vi "region-roll parameters-1.vi"() -> ()   [LabVIEW 2009]
panel:
  in  "Calculate 3":bool
  in  "Change_Max Diameter":dbl=108.0
  out "Region 3":dbl format="%_3g"
  out "Lap 3":dbl
  out "Set voltage value 2":dbl format="%_3g"
  out "Voltage difference value 2":dbl format="%_3g"
  in  "Speed-voltage constant 2":dbl=0.01
  out "Min Circular Speed 2":dbl format="%_3g"
  in  "Web Speed 2":dbl=90.0
  in  "Actual Diameter 2":dbl
  out "Max Circular Speed 2":dbl format="%_3g"
  in  "Max Diameter":dbl=108.0
  in  "Min Diameter":dbl=93.0
  in  "Diameter":dbl
  in  "Web Thickness 2":dbl=60.0
  out "Lap 2":dbl
  out "Region 2":dbl format="%_3g"
  out "Output voltage value 2":dbl=0.01 format="%.2g"
  in  "Calculate 2":bool
  in  "Calculate_auto":bool
  in  "Initial Min Diameter":dbl=93.0
  out "Output voltage value":dbl=0.01 format="%.2g"
  out "Set voltage value":dbl format="%_3g"
  out "Voltage difference value":dbl format="%_3g"
  in  "Speed-voltage constant":dbl=0.01
  out "Lap":dbl
  out "Region":dbl format="%_3g"
  in  "Web Thickness":dbl=60.0
  out "Min Circular Speed":dbl format="%_3g"
  out "Max Circular Speed":dbl format="%_3g"
  in  "Web Speed":dbl=90.0
  in  "Total length":dbl
  in  "Calculate":bool
  out "Actual Diameter":dbl
  in  "Change_Min Diameter":dbl=93.0
  # "m"
  # "mm"
  # "mm"
  # "µm"
  # "cm / min"
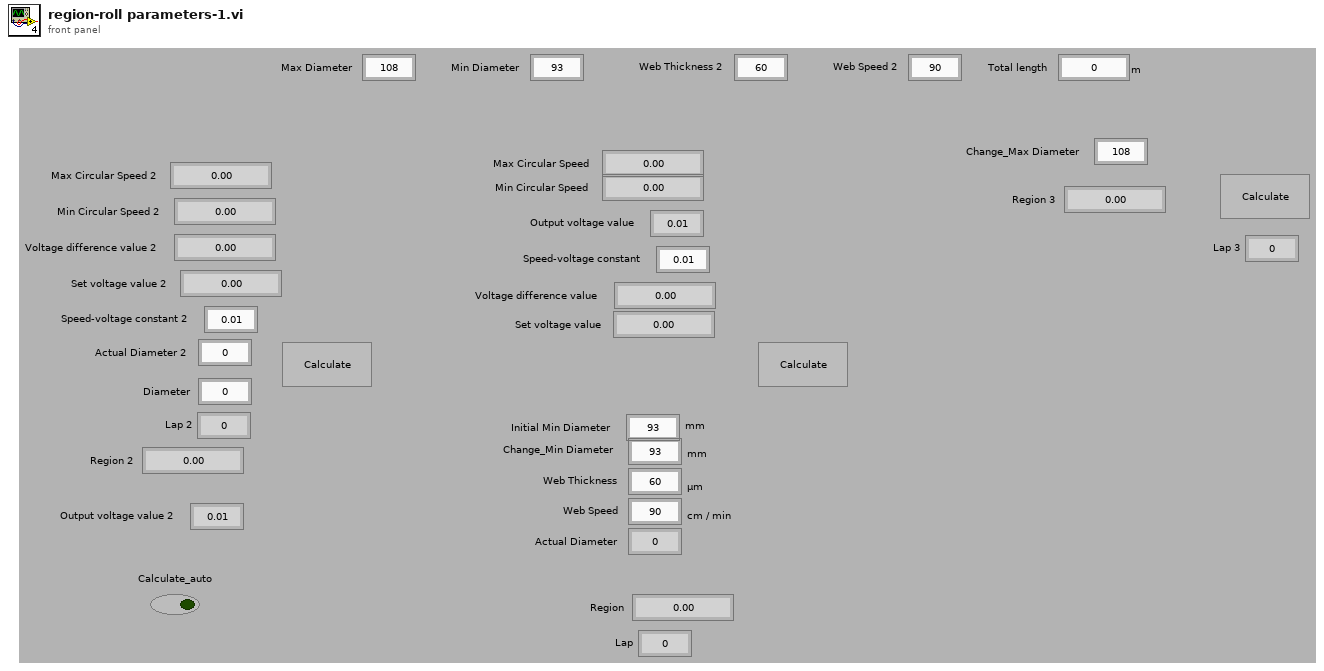
[diagram p1: front panel]
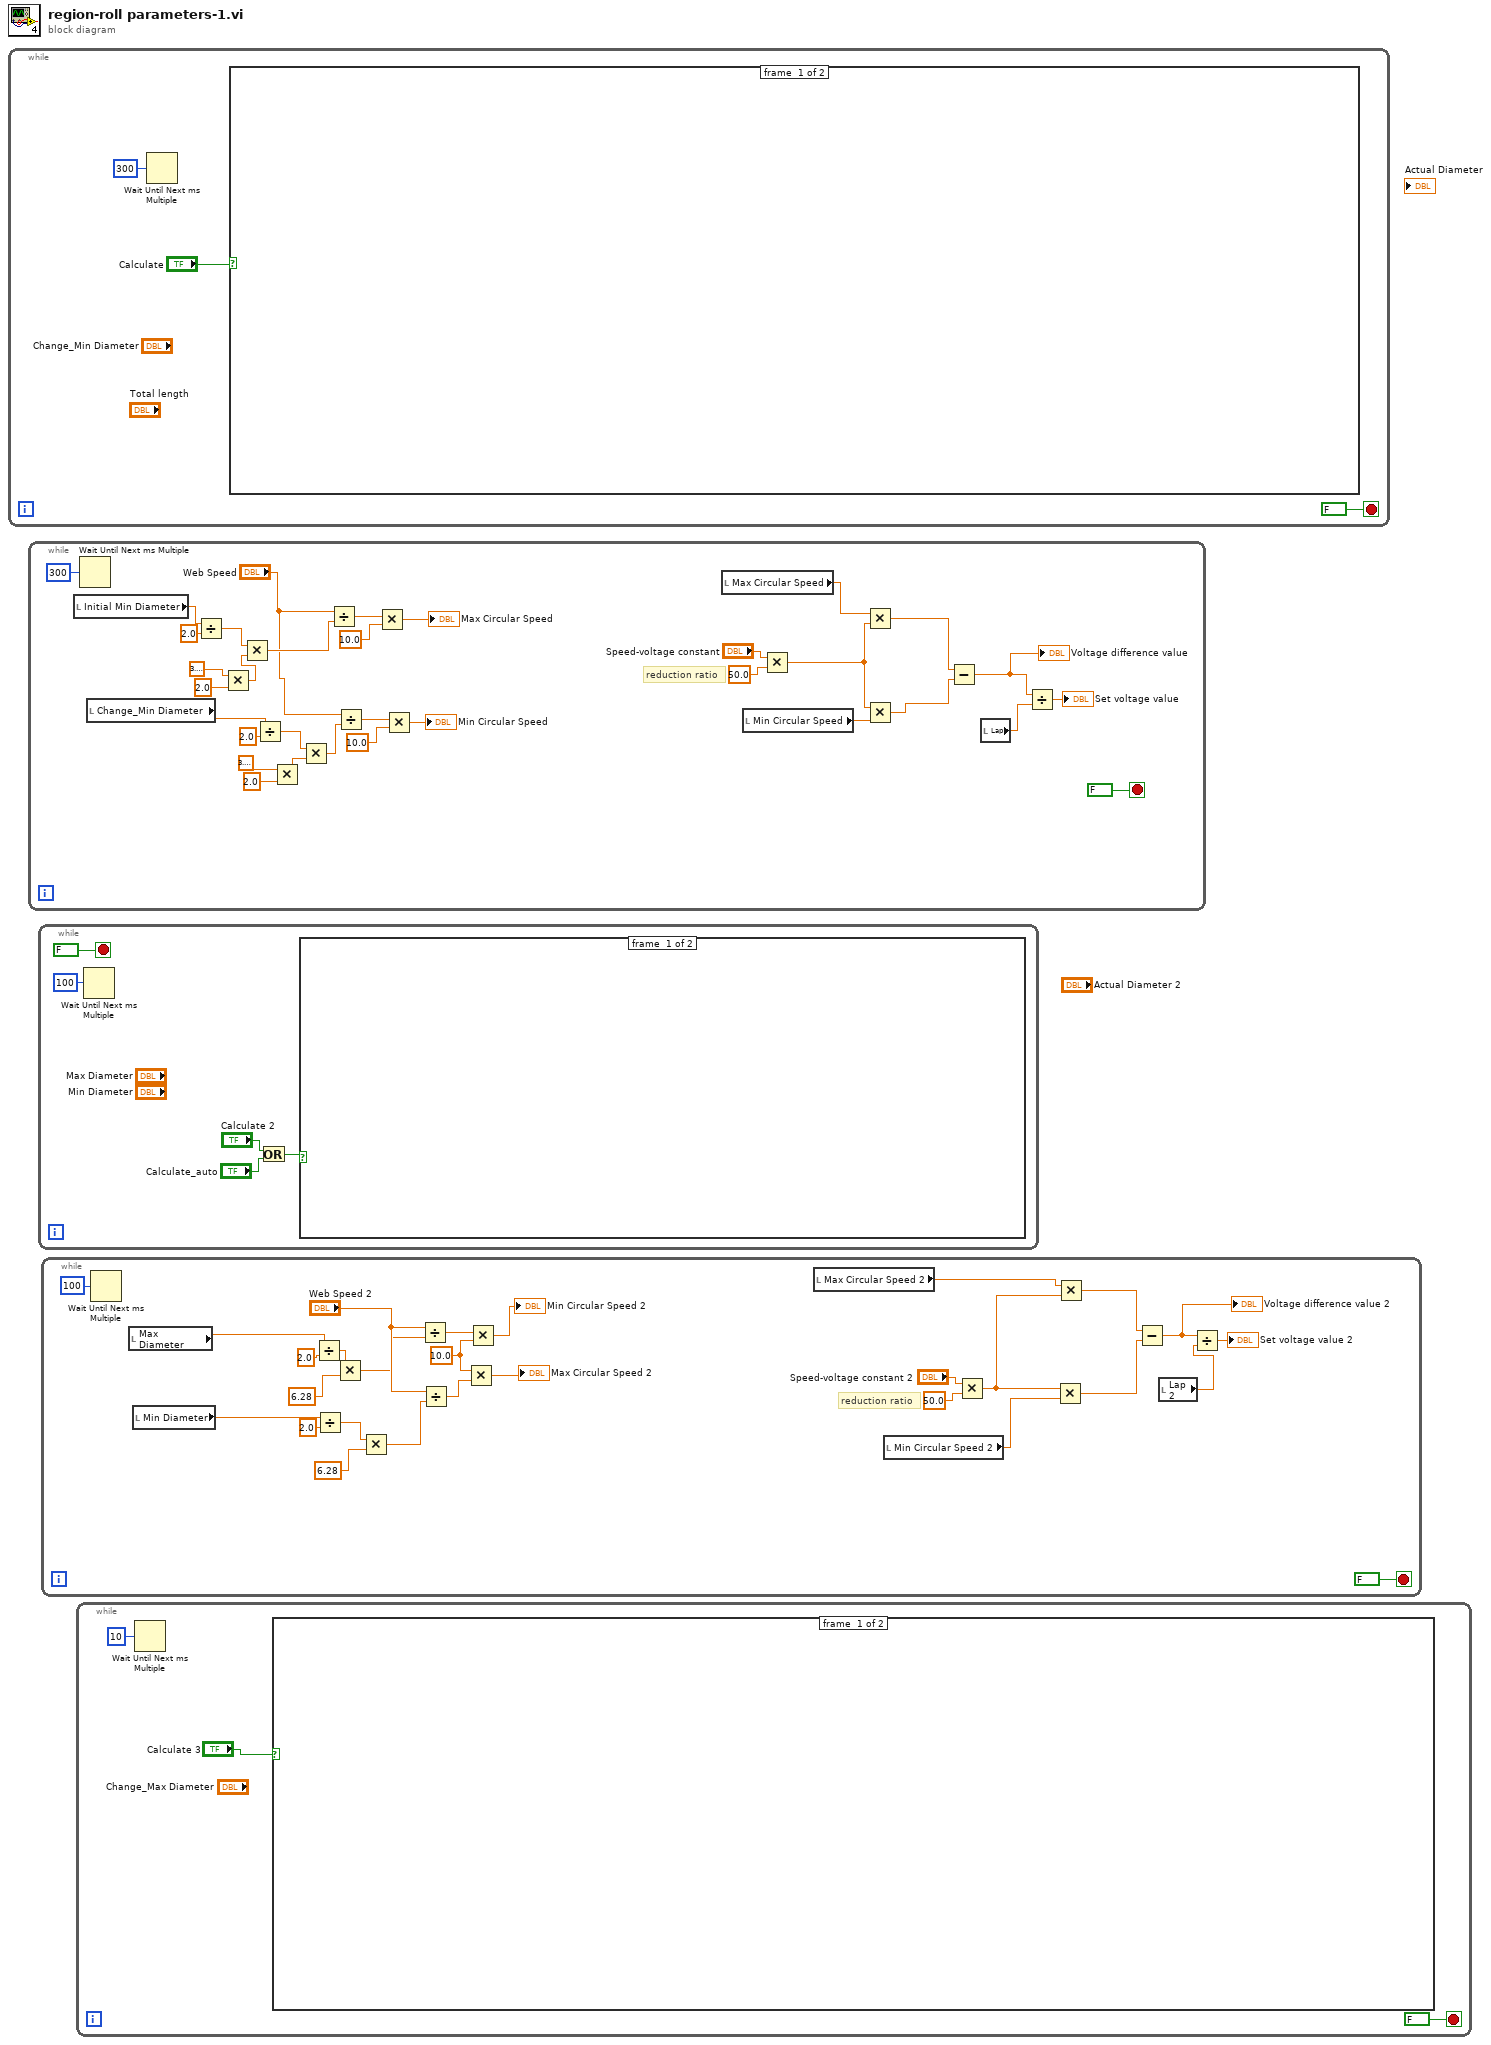
[diagram p0: block diagram]
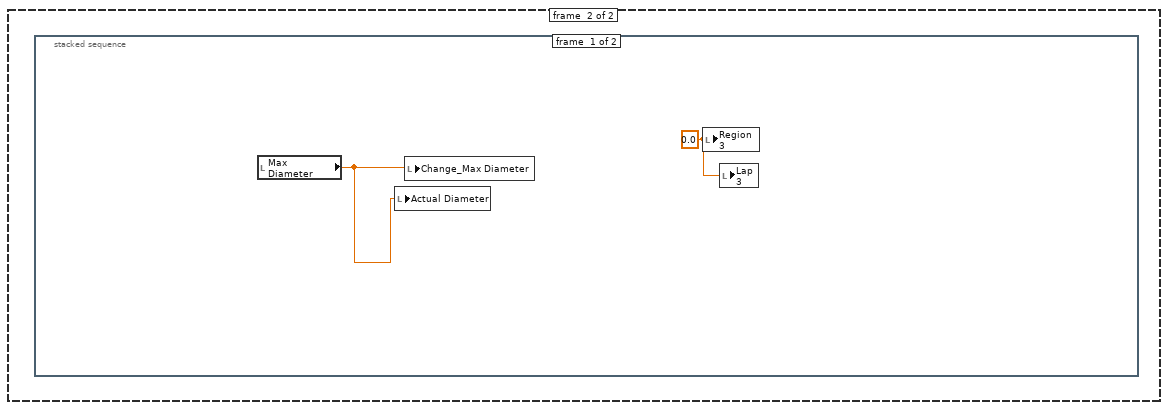
[diagram p2: hidden frame]
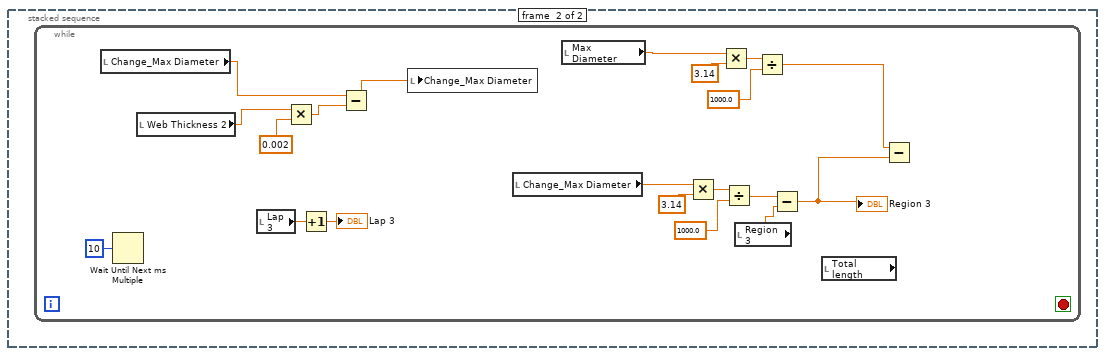
[diagram p3: hidden frame]
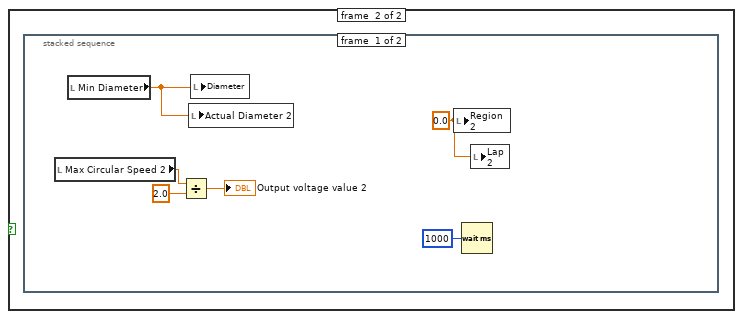
[diagram p4: hidden frame]
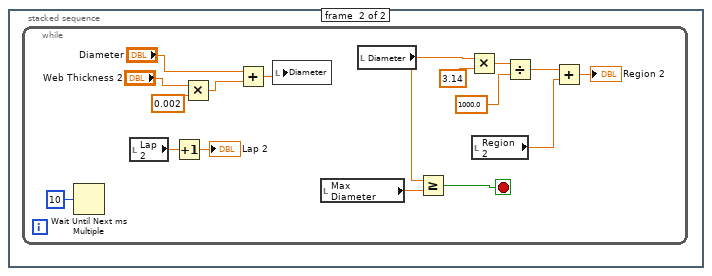
[diagram p5: hidden frame]
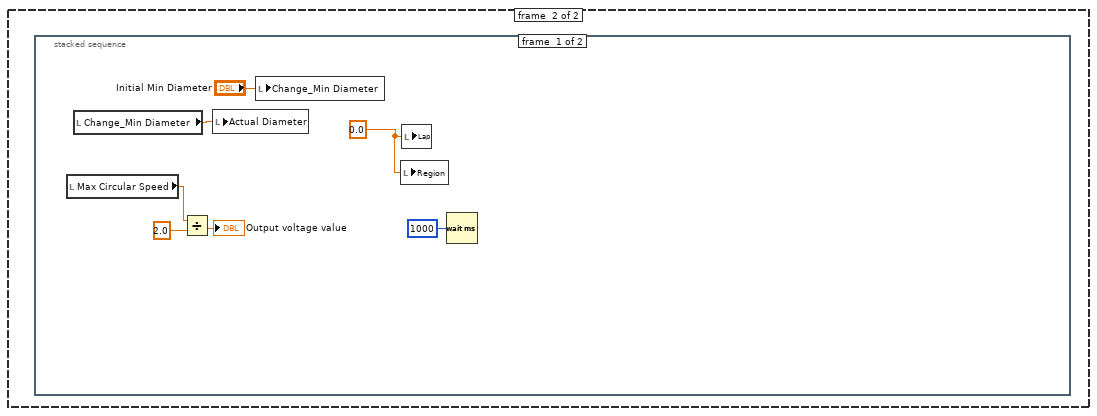
[diagram p6: hidden frame]
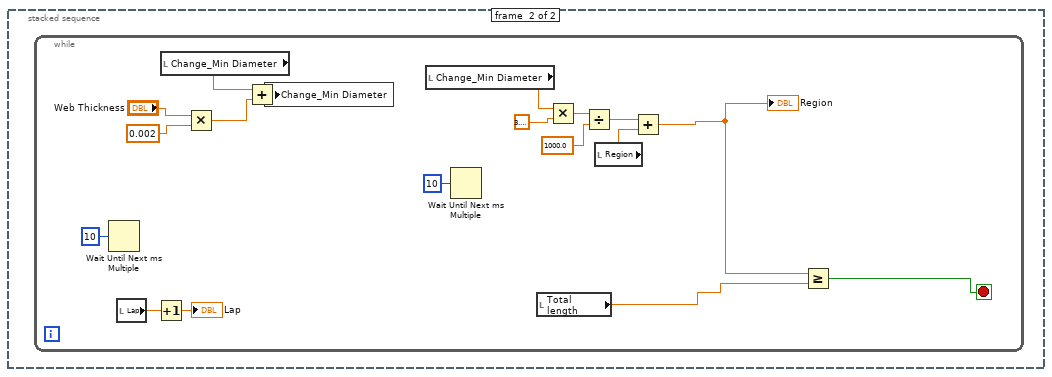
[diagram p7: hidden frame]
diagram:
  n1 = while {
    stop <- FALSE stop-if-true
    n2 = Wait Until Next ms Multiple(millisecond multiple=u32 300) -> ()  [unwired: 1 out]
    n3 = case shown="True" "Calculate" {
      frame #0 {
      }
      frame #1 {
        n4 = stacked-sequence {
          frame #0 {
            w4 = 0.0 ("Lap")
            n5 = local read "Max Circular Speed"() -> (w7:dbl)
            n6 = local read "Change_Min Diameter"() -> (w9:dbl)
            n7 = Divide(x=w7, y=2.0) -> (x/y=→"Output voltage value":dbl)
            n8 = local write "Actual Diameter"(w9) -> ()
            n9 = local write "Change_Min Diameter"("Initial Min Diameter") -> ()
            n10 = local write "Region"(w4) -> ()
            n11 = local write "Lap"(w4) -> ()
            n12 = Wait (ms)(milliseconds to wait=u32 1000) -> ()  [unwired: 1 out]
          }
          frame #1 {
            n13 = while {
              stop <- w20 stop-if-true
              n14 = Wait Until Next ms Multiple(millisecond multiple=u32 10) -> ()  [unwired: 1 out]
              n15 = local read "Lap"() -> (w23:dbl)
              n16 = Increment(x=w23) -> (x+1=→"Lap":dbl)
              n17 = local read "Change_Min Diameter"() -> (w27:dbl)
              n18 = Multiply(x="Web Thickness", y=0.002) -> (x*y=w26:dbl)
              n19 = Add(x=w27, y=w26) -> (x+y=w25:dbl)
              n20 = local write "Change_Min Diameter"(w25) -> ()
              n21 = local read "Change_Min Diameter"() -> (w17:dbl)
              n22 = Wait Until Next ms Multiple(millisecond multiple=u32 10) -> ()  [unwired: 1 out]
              n23 = local read "Total length"() -> (w11:dbl)
              n24 = Multiply(x=w17, y=3.141592653589793) -> (x*y=w18:dbl)
              n25 = Divide(x=w18, y=1000.0) -> (x/y=w19:dbl)
              n26 = local read "Region"() -> (w15:dbl)
              n27 = Add(x=w19, y=w15) -> (x+y=w12:dbl)
              "Region" <- w12
              n28 = Greater Or Equal?(x=w12, y=w11) -> (x >= y?=w20:bool)
            }
          }
        }
      }
    }
  }
  n29 = while {
    stop <- FALSE stop-if-true
    # "reduction ratio"
    n30 = local read "Initial Min Diameter"() -> (w29:dbl)
    n31 = Wait Until Next ms Multiple(millisecond multiple=u32 300) -> ()  [unwired: 1 out]
    n32 = local read "Change_Min Diameter"() -> (w30:dbl)
    n33 = Divide(x=w29, y=2.0) -> (x/y=w59:dbl)
    n34 = Multiply(x=3.141592653589793, y=2.0) -> (x*y=w45:dbl)
    n35 = Multiply(x=w59, y=w45) -> (x*y=w56:dbl)
    n36 = Divide(x=w30, y=2.0) -> (x/y=w51:dbl)
    n37 = Multiply(x=3.141592653589793, y=2.0) -> (x*y=w42:dbl)
    n38 = Multiply(x=w51, y=w42) -> (x*y=w54:dbl)
    n39 = Divide(x="Web Speed", y=w56) -> (x/y=w58:dbl)
    n40 = Divide(x="Web Speed", y=w54) -> (x/y=w52:dbl)
    n41 = Multiply(x=w58, y=10.0) -> (x*y=→"Max Circular Speed":dbl)
    n42 = Multiply(x=w52, y=10.0) -> (x*y=→"Min Circular Speed":dbl)
    n43 = local read "Max Circular Speed"() -> (w38:dbl)
    n44 = local read "Min Circular Speed"() -> (w37:dbl)
    n45 = Multiply(x="Speed-voltage constant", y=50.0) -> (x*y=w39:dbl)
    n46 = Multiply(x=w38, y=w39) -> (x*y=w36:dbl)
    n47 = Multiply(x=w39, y=w37) -> (x*y=w35:dbl)
    n48 = Subtract(x=w36, y=w35) -> (x-y=w32:dbl)
    "Voltage difference value" <- w32
    n49 = local read "Lap"() -> (w33:dbl)
    n50 = Divide(x=w32, y=w33) -> (x/y=→"Set voltage value":dbl)
  }
  n51 = while {
    stop <- FALSE stop-if-true
    n52 = Wait Until Next ms Multiple(millisecond multiple=u32 100) -> ()  [unwired: 1 out]
    n53 = Or(x="Calculate 2", y="Calculate_auto") -> (x .or. y?=w64:bool)
    n54 = case shown="True" w64 {
      frame #0 {
      }
      frame #1 {
        n55 = stacked-sequence {
          frame #0 {
            w71 = 0.0 ("Region")
            n56 = local read "Max Circular Speed 2"() -> (w68:dbl)
            n57 = local read "Min Diameter"() -> (w67:dbl)
            n58 = Divide(x=w68, y=2.0) -> (x/y=→"Output voltage value 2":dbl)
            n59 = local write "Actual Diameter 2"(w67) -> ()
            n60 = local write "Diameter"(w67) -> ()
            n61 = local write "Region 2"(w71) -> ()
            n62 = Wait (ms)(milliseconds to wait=u32 1000) -> ()  [unwired: 1 out]
            n63 = local write "Lap 2"(w71) -> ()
          }
          frame #1 {
            n64 = while {
              stop <- w76 stop-if-true
              n65 = Wait Until Next ms Multiple(millisecond multiple=u32 10) -> ()  [unwired: 1 out]
              n66 = local read "Lap 2"() -> (w73:dbl)
              n67 = Increment(x=w73) -> (x+1=→"Lap 2":dbl)
              n68 = Multiply(x="Web Thickness 2", y=0.002) -> (x*y=w87:dbl)
              n69 = Add(x="Diameter", y=w87) -> (x+y=w79:dbl)
              n70 = local write "Diameter"(w79) -> ()
              n71 = local read "Max Diameter"() -> (w78:dbl)
              n72 = local read "Diameter"() -> (w77:dbl)
              n73 = Greater Or Equal?(x=w77, y=w78) -> (x >= y?=w76:bool)
              n74 = Multiply(x=w77, y=3.14) -> (x*y=w81:dbl)
              n75 = local read "Region 2"() -> (w85:dbl)
              n76 = Divide(x=w81, y=1000.0) -> (x/y=w84:dbl)
              n77 = Add(x=w84, y=w85) -> (x+y=→"Region 2":dbl)
            }
          }
        }
      }
    }
  }
  n78 = while {
    stop <- FALSE stop-if-true
    w113 = 10.0 ("y")
    # "reduction ratio"
    n79 = Wait Until Next ms Multiple(millisecond multiple=u32 100) -> ()  [unwired: 1 out]
    n80 = local read "Max Diameter"() -> (w103:dbl)
    n81 = local read "Min Diameter"() -> (w102:dbl)
    n82 = Divide(x=w103, y=2.0) -> (x/y=w108:dbl)
    n83 = Divide(x=w102, y=2.0) -> (x/y=w107:dbl)
    n84 = Multiply(x=w108, y=6.28) -> (x*y=w109:dbl)
    n85 = Multiply(x=w107, y=6.28) -> (x*y=w106:dbl)
    n86 = Divide(x="Web Speed 2", y=w109) -> (x/y=w115:dbl)
    n87 = Divide(x="Web Speed 2", y=w106) -> (x/y=w114:dbl)
    n88 = Multiply(x=w113, y=w114) -> (x*y=→"Max Circular Speed 2":dbl)
    n89 = Multiply(x=w115, y=w113) -> (x*y=→"Min Circular Speed 2":dbl)
    n90 = local read "Max Circular Speed 2"() -> (w99:dbl)
    n91 = local read "Min Circular Speed 2"() -> (w97:dbl)
    n92 = Multiply(x="Speed-voltage constant 2", y=50.0) -> (x*y=w98:dbl)
    n93 = Multiply(x=w98, y=w97) -> (x*y=w93:dbl)
    n94 = Multiply(x=w99, y=w98) -> (x*y=w94:dbl)
    n95 = Subtract(x=w94, y=w93) -> (x-y=w96:dbl)
    "Voltage difference value 2" <- w96
    n96 = local read "Lap 2"() -> (w92:dbl)
    n97 = Divide(x=w96, y=w92) -> (x/y=→"Set voltage value 2":dbl)
  }
  n98 = while {
    stop <- FALSE stop-if-true
    n99 = Wait Until Next ms Multiple(millisecond multiple=u32 10) -> ()  [unwired: 1 out]
    n100 = case shown="True" "Calculate 3" {
      frame #0 {
      }
      frame #1 {
        n101 = stacked-sequence {
          frame #0 {
            w122 = 0.0 ("Region")
            n102 = local read "Max Diameter"() -> (w121:dbl)
            n103 = local write "Actual Diameter"(w121) -> ()
            n104 = local write "Change_Max Diameter"(w121) -> ()
            n105 = local write "Region 3"(w122) -> ()
            n106 = local write "Lap 3"(w122) -> ()
          }
          frame #1 {
            n107 = while {
              stop <- _ stop-if-true
              n108 = local read "Change_Max Diameter"() -> (w133:dbl)
              n109 = Wait Until Next ms Multiple(millisecond multiple=u32 10) -> ()  [unwired: 1 out]
              n110 = local read "Web Thickness 2"() -> (w141:dbl)
              n111 = local read "Lap 3"() -> (w139:dbl)
              n112 = Multiply(x=w141, y=0.002) -> (x*y=w142:dbl)
              n113 = Increment(x=w139) -> (x+1=→"Lap 3":dbl)
              n114 = Subtract(x=w133, y=w142) -> (x-y=w132:dbl)
              n115 = local write "Change_Max Diameter"(w132) -> ()
              n116 = local read "Change_Max Diameter"() -> (w130:dbl)
              n117 = local read "Max Diameter"() -> (w126:dbl)
              n118 = Multiply(x=w130, y=3.14) -> (x*y=w137:dbl)
              n119 = Multiply(x=w126, y=3.14) -> (x*y=w128:dbl)
              n120 = Divide(x=w137, y=1000.0) -> (x/y=w135:dbl)
              n121 = local read "Region 3"() -> (w134:dbl)
              n122 = Divide(x=w128, y=1000.0) -> (x/y=w125:dbl)
              n123 = Subtract(x=w135, y=w134) -> (x-y=w124:dbl)
              "Region 3" <- w124
              n124 = local read "Total length"() -> ()  [unwired: 1 out]
              n125 = Subtract(x=w125, y=w124) -> ()  [unwired: 1 out]
            }
          }
        }
      }
    }
  }
